vi "Build Stim Update Cmd_new.vi"(5 "Stimulator":T1={"Stim Open Data"={"Name"="", "Mode"=enum."LIVE", "Visa Timeout"=0}, "Stim Init Data"={"Frequency"=0.0, "N Factor"=0, "D/T Int"=0.0, "Active Channels"=[FALSE], "LF Channels"=[]}, "Stim Update Data"={"Pulse Mode"=[], "Current"=[], "Pulse Dur"=[]}, "Stim Status"={"Open"=FALSE, "On"=FALSE}}) -> (1 "Command":T9, 2 "Stimulator":T1={"Stim Open Data"={"Name"="", "Mode"=enum."LIVE", "Visa Timeout"=0}, "Stim Init Data"={"Frequency"=0.0, "N Factor"=0, "D/T Int"=0.0, "Active Channels"=[FALSE], "LF Channels"=[]}, "Stim Update Data"={"Pulse Mode"=[], "Current"=[], "Pulse Dur"=[]}, "Stim Status"={"Open"=FALSE, "On"=FALSE}})   [LabVIEW 2019]
uses:
  Data Type Defs/Pulse Mode (array).ctl
  Controls/Pulse Duration Array.ctl
  Controls/Stim Current Array.ctl
  Data Type Defs/Stimulator.ctl
  Data Type Defs/Stim Open Data.ctl
  Data Type Defs/Stim Init Data.ctl
  Data Type Defs/Stim Update Data.ctl
  Data Type Defs/Stim Status.ctl
panel:
  out "Current Array":T7
  out "Pulse Duration Array":T8
  out "Channel Number":i32
  out "Active Channels":bool[](array[boolean])
  out "Mode Array":T5
  # "This VI implements the Channel list mode update command from the Hasomed RehaStim."
  # "Inputs\nStim Frequency - the main frequency of stimulation in Hz.  The Hasomed Rehastim Science Mode documentation defines this as 1/t1.  We typically use 40 Hz for FES applications.\nGroup Time - for multi-pulse stimulation, enter the inter-pulse interval (aka pulse repetition interval) here.  We typically use single pulses (Group Time = 0).\nN factor - the factor by which t1 is multiplied to get the \"Low Frequency\" channel period.  This is optional - we typically do not use it.\nChannel Stim Boolean Array - defines the active channels (up to 8).\nChannel LF Boolean Array - defines the channels for which \"low frequency\" will be used.  Low frequency is defined as 1/(N_factor * Stim_Frequency).\n\nOutputs\nChannel List Mode Init Cmd String - the string of Hex numbers representing the final command."
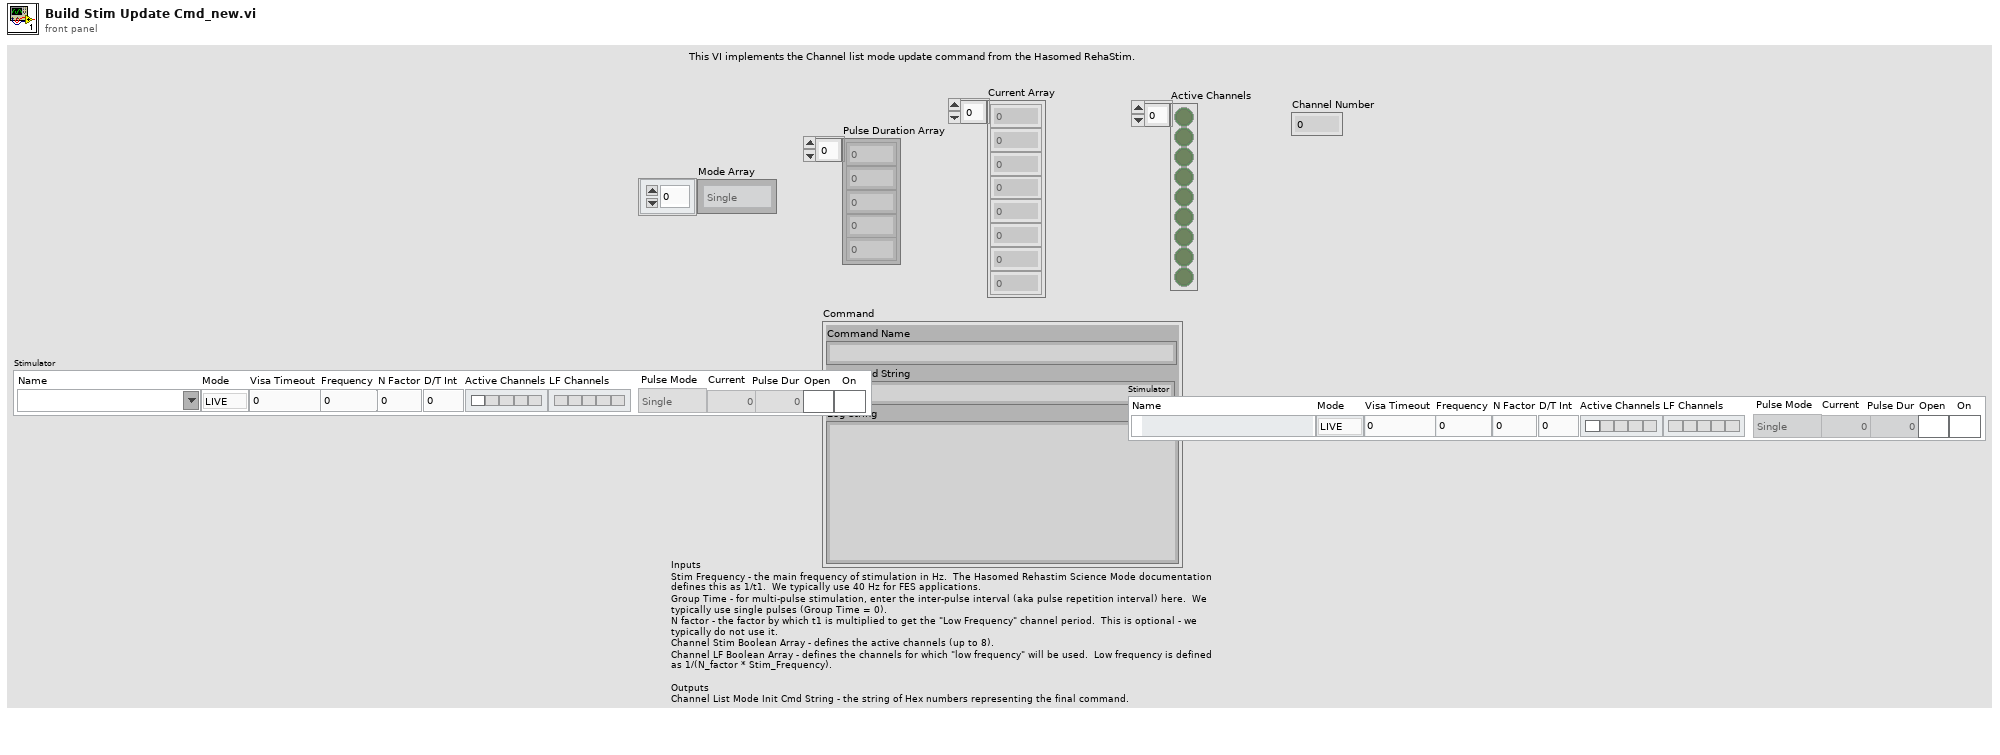
[diagram p1: front panel]
types:
  T1 = typedef "Stimulator.ctl" = cluster{"Stim Open Data":T2, "Stim Init Data":T3, "Stim Update Data":T4, "Stim Status":T6}
  T2 = typedef "Stim Open Data.ctl" = cluster{"Name":refnum<visa-resource-name>, "Mode":enum16{"LIVE", "SIM"}, "Visa Timeout":u32}
  T3 = typedef "Stim Init Data.ctl" = cluster{"Frequency":dbl, "N Factor":u8, "D/T Int":dbl, "Active Channels":bool[], "LF Channels":bool[]}
  T4 = typedef "Stim Update Data.ctl" = cluster{"Pulse Mode":T5, "Current":u32[], "Pulse Dur":u32[]}
  T5 = typedef "Pulse Mode (array).ctl" = enum16{"Single", "Doublet", "Triplet"}[]
  T6 = typedef "Stim Status.ctl" = cluster{"Open":bool, "On":bool}
  T7 = typedef "Stim Current Array.ctl" = u8[]
  T8 = typedef "Pulse Duration Array.ctl" = u32[]
  T9 = cluster{"Command Name":string, "Command String":string, "Log String":string}
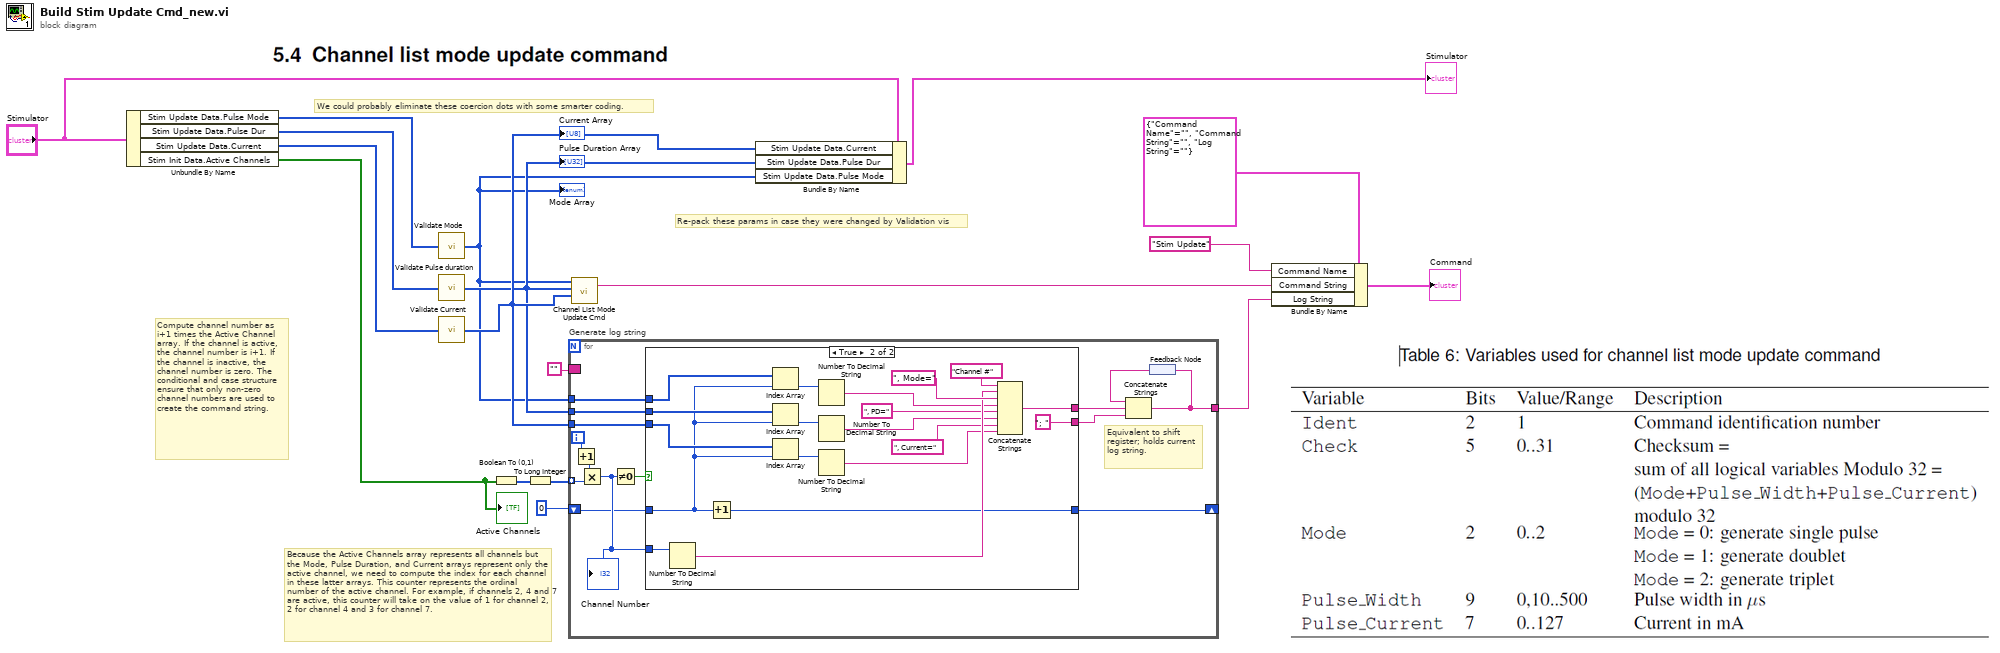
[diagram p0: block diagram]
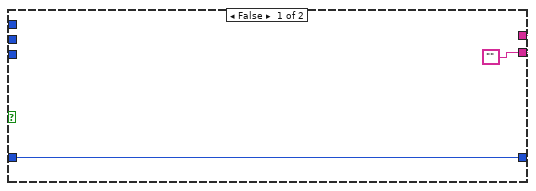
[diagram p2: hidden frame]
diagram:
  # "We could probably eliminate these coercion dots with some smarter coding."
  # "Re-pack these params in case they were changed by Validation vis"
  # "Because the Active Channels array represents all channels but the Mode, Pulse Duration, and Current arrays represent only the active channel, we need to compute the index for each channel in these latter arrays. This counter represents the ordinal number of the active channel. For example, if channels 2, 4 and 7 are active, this counter will take on the value of 1 for channel 2, 2 for channel 4 and 3 for channel 7."
  # "Compute channel number as i+1 times the Active Channel array. If the channel is active, the channel number is i+1. If the channel is inactive, the channel number is zero. The conditional and case structure ensure that only non-zero channel numbers are used to create the command string."
  n1 = Unbundle By Name("Stimulator") -> ("Stim Update Data.Pulse Mode"=w7:T5, "Stim Update Data.Pulse Dur"=w6:u32[], "Stim Update Data.Current"=w8:u32[], "Stim Init Data.Active Channels"=w18:bool[])
  "Active Channels" <- w18
  n2 = call "Validate Mode.vi"("Mode Array"=w7) -> ("Mode"=w3:i16[])
  "Mode Array" <- w3
  n3 = call "Validate Pulse duration.vi"("Pulse Duration"=w6) -> ("Pulse Duration"=w4:u32[])
  "Pulse Duration Array" <- w4
  n4 = call "Validate Current.vi"("Current Array"=w8) -> ("Current Out"=w5:u8[])
  "Current Array" <- w5
  n5 = Boolean To (0,1)(Boolean=w18) -> (0, 1=w17:i16[])
  n6 = To Long Integer(number=w17) -> (32bit integer=w16:i32[])
  n7 = for "Generate log string" {
    tunnel: w16 -> [w21] mode=indexing
    tunnel: w3 -> [w30]
    tunnel: w5 -> [w29]
    tunnel: w4 -> [w27]
    tunnel: [w25] -> w12
    border: "" -> [_]
    shift-right: [w19] -> _
    shift-left: 0 -> [w20]
    i -> [w32]
    # "Equivalent to shift register; holds current log string."
    n8 = Increment(x=w32) -> (x+1=w22:i32)
    n9 = Multiply(x=w22, y=w21) -> (x*y=w28:i32)
    "Channel Number" <- w28
    n10 = Not Equal To 0?(x=w28) -> (x != 0?=w31:bool)
    n11 = case shown="True" w31 {
      tunnel: w30 -> [_ w53]
      tunnel: w29 -> [_ w52]
      tunnel: w28 -> [_ w48]
      tunnel: w27 -> [_ w49]
      tunnel: [w34 w38] -> w23
      tunnel: [w34 "; "] -> w24
      tunnel: w20 -> [w33 w36]
      tunnel: [w33 w35] -> w19
      frame False {
        w34 = ""
      }
      frame True {
        n12 = Number To Decimal String(number=w48) -> (decimal integer string=w45:string)  [unwired: 1 in]
        n13 = Increment(x=w36) -> (x+1=w35:i32)
        n14 = Index Array(array=w53, index=w36) -> (element=w44:i16)
        n15 = Index Array(array=w49, index=w36) -> (element=w47:u32)
        n16 = Index Array(array=w52, index=w36) -> (element=w51:u8)
        n17 = Number To Decimal String(number=w44) -> (decimal integer string=w43:string)  [unwired: 1 in]
        n18 = Number To Decimal String(number=w47) -> (decimal integer string=w41:string)  [unwired: 1 in]
        n19 = Number To Decimal String(number=w51) -> (decimal integer string=w39:string)  [unwired: 1 in]
        n20 = Concatenate Strings("Channel #", w45, ", Mode=", w43, ", PD=", w41, ", Current=", w39) -> (w38:string)
      }
    }
    n21 = feedback #1() -> (w26:string)
    n22 = Concatenate Strings(w26, w23, w24) -> (w25:string)
    n23 = feedback-in #1(w25) -> ()
  }
  n24 = call "Channel List Mode Update Cmd.vi"("Current Array"=w5, "Pulse Duration"=w4, "Mode Array"=w3) -> ("Channel List Mode Init Cmd String"=w13:string)  [unwired: 2 in]
  n25 = Bundle By Name(cluster="Stimulator", "Stim Update Data.Current"=w5, "Stim Update Data.Pulse Dur"=w4, "Stim Update Data.Pulse Mode"=w3) -> (→"Stimulator":T1)
  n26 = Bundle By Name(cluster=T9 {"Command Name"="", "Command String"="", "Log String"=""}, "Command Name"="Stim Update", "Command String"=w13, "Log String"=w12) -> (→"Command":T9)
